vi "balanzaLabview.vi"() -> ()   [LabVIEW 2017]
uses:
  <vilib>/Instr/_visa.llb/VISA Configure Serial Port (Instr).vi
panel:
  in  "Unit Select":string(combo)
  out "Waveform Chart":i32(graph)
  out "Numeric":dbl
  out "string":string
  in  "?":bool
  in  "?":bool
  in  "Frenar Modo Activo":bool
  in  "Mode Select":string(combo)
  in  "Reiniciar":bool
  in  "Enviar":bool
  in  "Para modos con Intervalo":string
  out "buffer":string
  in  "VISA resource name":refnum<visa-resource-name>
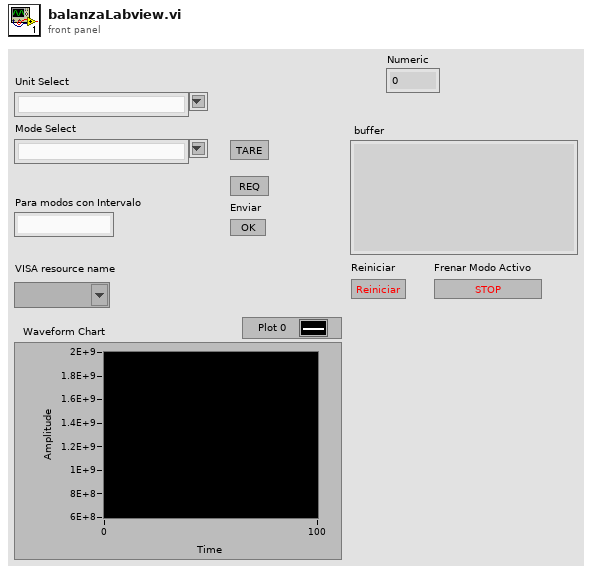
[diagram p1: front panel]
types:
  T1 = enum8{"Enabled", "Disabled", "Disabled and Grayed Out"}
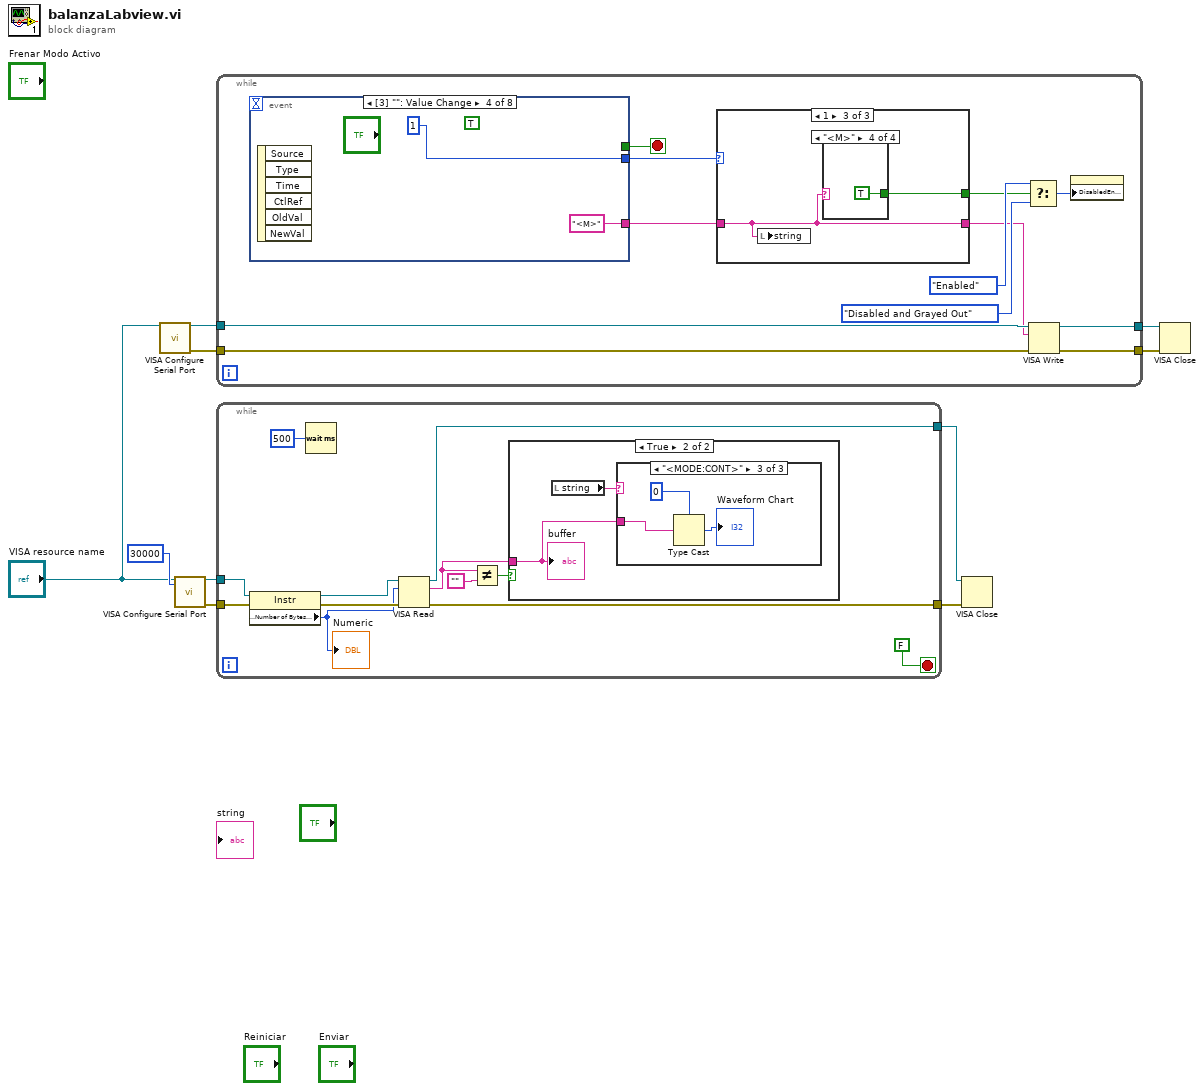
[diagram p0: block diagram]
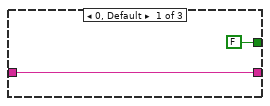
[diagram p5: hidden frame]
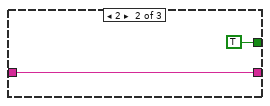
[diagram p6: hidden frame]
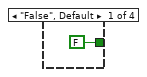
[diagram p7: hidden frame]
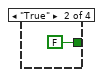
[diagram p8: hidden frame]
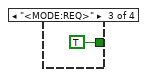
[diagram p9: hidden frame]
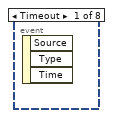
[diagram p10: hidden frame]
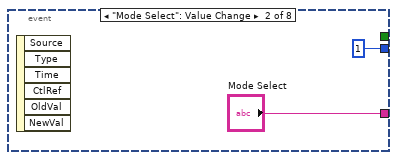
[diagram p11: hidden frame]
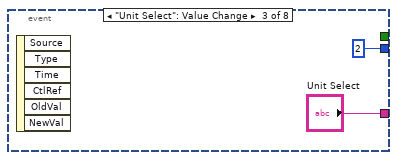
[diagram p12: hidden frame]
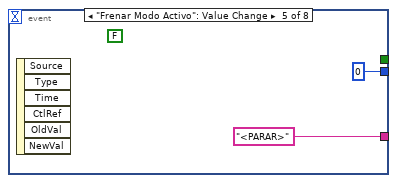
[diagram p13: hidden frame]
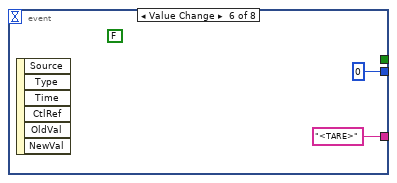
[diagram p14: hidden frame]
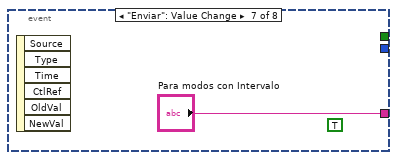
[diagram p15: hidden frame]
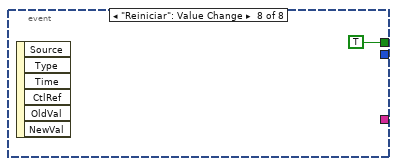
[diagram p16: hidden frame]
diagram:
  n1 = call-poly "VISA Configure Serial Port"("VISA resource name"="VISA resource name") -> ("VISA resource name out"=w10:refnum<visa-resource-name>, "error out"=w9:errorcluster)  [unwired: 13 in]
  n2 = call-poly "VISA Configure Serial Port"("VISA resource name"="VISA resource name", "timeout (10sec)"=u32 30000) -> ("VISA resource name out"=w7:refnum<visa-resource-name>, "error out"=w6:errorcluster)  [unwired: 12 in]
  n3 = while {
    tunnel: w10 -> [w21]
    tunnel: w9 -> [w22]
    tunnel: [w19] -> w4
    tunnel: [w18] -> w3
    stop <- w20 stop-if-true
    n4 = event shown="[3] \"\": Value Change" {
      selector: _ -> [_ _ _ _ _ _ _ _]
      dyn-events: _ -> [_ _ _ _ _ _ _ _]
      timeout: _ -> [_ _ _ _ _ _ _ _]
      tunnel: [_ "Mode Select" "Unit Select" "<M>" "<PARAR>" "<TARE>" "Para modos con Intervalo" _] -> w13
      tunnel: [_ _ _ _ _ _ _ TRUE] -> w20
      tunnel: [_ 1 2 1 0 0 _ _] -> w11
      event Timeout {
        n5 = event-data() -> ()  [unwired: 1 in, 3 out]
      }
      event "Mode Select": Value Change {
        n6 = event-data() -> ()  [unwired: 1 in, 6 out]
      }
      event "Unit Select": Value Change {
        n7 = event-data() -> ()  [unwired: 1 in, 6 out]
      }
      event Value Change {
        (unwired) TRUE
        n8 = event-data() -> ()  [unwired: 1 in, 6 out]
      }
      event "Frenar Modo Activo": Value Change {
        (unwired) FALSE
        n9 = event-data() -> ()  [unwired: 1 in, 6 out]
      }
      event Value Change {
        (unwired) FALSE
        n10 = event-data() -> ()  [unwired: 1 in, 6 out]
      }
      event "Enviar": Value Change {
        (unwired) TRUE
        n11 = event-data() -> ()  [unwired: 1 in, 6 out]
      }
      event "Reiniciar": Value Change {
        n12 = event-data() -> ()  [unwired: 1 in, 6 out]
      }
    }
    n13 = case shown="1" w11 {
      tunnel: [FALSE TRUE w28] -> w14
      tunnel: w13 -> [w24 w25 w27]
      tunnel: [w24 w25 w27] -> w12
      frame 0, Default {
      }
      frame 2 {
      }
      frame 1 {
        n14 = local write "string"(w27) -> ()
        n15 = case shown="\"<M>\"" w27 {
          tunnel: [FALSE FALSE TRUE TRUE] -> w28
          frame "False", Default {
          }
          frame "True" {
          }
          frame "<MODE:REQ>" {
          }
          frame "<M>" {
          }
        }
      }
    }
    n16 = Select(t=T1."Enabled" ("Disabled"), s=w14, f=T1."Disabled and Grayed Out" ("Disabled")) -> (s? t:f=w17:T1)
    n17 = VISA Write(VISA resource name=w21, write buffer=w12, error in (no error)=w22) -> (VISA resource name out=w19:refnum<visa-resource-name>, error out=w18:errorcluster)  [unwired: 1 out]
    n18 = property class="Bool (strict)"("DisabledEnum"=w17) -> ()  [unwired: 2 in, 2 out]
  }
  n19 = while {
    tunnel: w7 -> [w53]
    tunnel: w6 -> [w52]
    tunnel: [w55] -> w2
    tunnel: [w54] -> w1
    stop <- FALSE stop-if-true
    n20 = property class="Instr"(reference=w53, error in=w52) -> (reference out=w51:refnum<visa-resource-name>, error out=w50:errorcluster, "Serial Settings:Number of Bytes at Serial Port"=w48:u32)
    "Numeric" <- w48
    n21 = Wait (ms)(milliseconds to wait=u32 500) -> ()  [unwired: 1 out]
    n22 = VISA Read(VISA resource name=w51, byte count=w48, error in (no error)=w50) -> (VISA resource name out=w55:refnum<visa-resource-name>, read buffer=w45:string, error out=w54:errorcluster)  [unwired: 1 out]
    n23 = Not Equal?(x=w45, y="") -> (x != y?=w46:bool)
    n24 = case shown="True" w46 {
      tunnel: w45 -> [_ w57]
      frame False {
      }
      frame True {
        n25 = local read "string"() -> (w58:string)
        n26 = case shown="\"<MODE:CONT>\"" w58 {
          tunnel: w57 -> [_ _ w59]
          frame "False", Default {
          }
          frame "True" {
          }
          frame "<MODE:CONT>" {
            n27 = Type Cast(type=0, x=w59) -> (*(type *) &x=→"Waveform Chart":i32)
          }
        }
        "buffer" <- w57
      }
    }
  }
  n28 = VISA Close(VISA resource name=w2, error in (no error)=w1) -> ()  [unwired: 1 out]
  n29 = VISA Close(VISA resource name=w4, error in (no error)=w3) -> ()  [unwired: 1 out]
